vi "Waveform In Volatile.vi"(8 "error in (no error)":errorcluster, 9 "Arbitrary Waveform Name":string, 10 "Channel (1: 1)":i32(ring)=1 items=["1"=1, "2"=2], 11 "VISA resource name":refnum<visa-resource-name>) -> (0 "error out":errorcluster, 2 "Wave In Volatile?":bool, 3 "VISA resource name out":refnum<visa-resource-name>)   [LabVIEW 2016, in "Agilent 3352X Series.lvlib"]
doc: "Checks if specific Arb Waveform already loaded into volatile memory."
uses:
  Agilent 3352X Series.lvlib
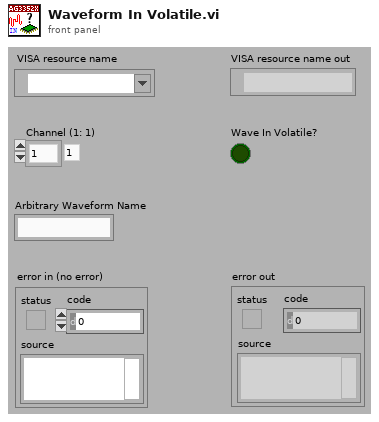
[diagram p1: front panel]
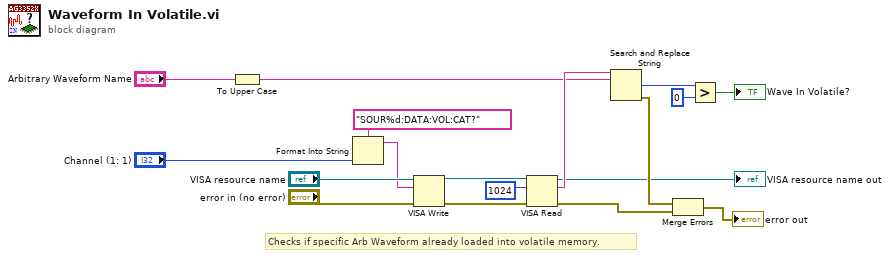
[diagram p0: block diagram]
diagram:
  # "Checks if specific Arb Waveform already loaded into volatile memory."
  n1 = To Upper Case(1:"Arbitrary Waveform Name") -> (0:w1:string)
  n2 = Format Into String(format string="SOUR%d:DATA:VOL:CAT?", "Channel (1: 1)") -> (resulting string=w14:string)  [unwired: 2 in, 1 out]
  n3 = VISA Write(VISA resource name="VISA resource name", write buffer=w14, error in (no error)="error in (no error)") -> (VISA resource name out=w13:refnum<visa-resource-name>, error out=w12:errorcluster)  [unwired: 1 out]
  n4 = VISA Read(VISA resource name=w13, byte count=u32 1024, error in (no error)=w12) -> (VISA resource name out=→"VISA resource name out":refnum<visa-resource-name>, read buffer=w10:string, error out=w5:errorcluster)  [unwired: 1 out]
  n5 = Search and Replace String(input string=w10, search string=w1) -> (number of replacements=w9:i32, error out=w6:errorcluster)  [unwired: 1 in, 7 out]
  n6 = Merge Errors(w6, w5) -> (→"error out":errorcluster)
  n7 = Greater?(x=w9, y=0) -> (0:→"Wave In Volatile?":bool)
